vi "IPX_HTTP_Read_DI.vi"(8 "Error In":errorcluster, 9 "Voie":u16(ring) items=["1", "2", "3", "4", "5", "6", "7", "8"], 10 "Port (80-8000)":dbl=80.0, 11 "IP adress (XXX.XXX.XXX.XXX)":string) -> (0 "Error Out":errorcluster, 2 "Value":i16)   [LabVIEW 2014, in "IPX_HTTP.lvlib"]
uses:
  IPX_HTTP.lvlib
panel:
  # "Lecture des DI de la carte IPX via la lecture du status.xml"
  # "Digital Input"
  # "Please visit http://www.OpenG.org to learn about the\nOpen Source LabVIEW software movement.\n\nNOTICE -- YOU MUST LEAVE THIS NOTICE IN PLACE.  PER THE TERMS OF THE LICENSE BELOW, YOU MAY SUBLICENSE THIS SOFTWARE\nIN ANY WAY THAT DOES NOT CONFLICT WITH THIS LICENSE.\n\n### BSD License (http://www.opensource.org/licenses/bsd-license.php) Begin ###\n\nCopyright (c) 2014, Emmanuel Landrivon <emmanuel.landrivon@ircelyon.univ-lyon1.fr>\nFlorian Chapon <florian.chapon@ircelyon.univ-lyon1.fr\n\n\nAll rights reserved.\n\nRedistribution and use in source and binary forms, with or without modification, are permitted provided that the following conditions are met:\n\n    * Redistributions of source code must retain the above copyright notice, this list of conditions and the following disclaimer.\n    * Redistributions in binary form must reproduce the above copyright notice, this list of conditions and the following disclaimer in the\n       documentation and/or other materials provided with the distribution.\n  \nTHIS SOFTWARE IS PROVIDED BY THE COPYRIGHT HOLDERS AND CONTRIBUTORS \"AS IS\" AND ANY EXPRESS OR IMPLIED WARRANTIES,\nINCLUDING, BUT NOT LIMITED TO, THE IMPLIED WARRANTIES OF MERCHANTABILITY AND FITNESS FOR A PARTICULAR PURPOSE ARE\nDISCLAIMED. IN NO EVENT SHALL THE COPYRIGHT OWNER OR CONTRIBUTORS BE LIABLE FOR ANY DIRECT, INDIRECT, INCIDENTAL,\nSPECIAL, EXEMPLARY, OR CONSEQUENTIAL DAMAGES (INCLUDING, BUT NOT LIMITED TO, PROCUREMENT OF SUBSTITUTE GOODS OR\nSERVICES; LOSS OF USE, DATA, OR PROFITS; OR BUSINESS INTERRUPTION) HOWEVER CAUSED AND ON ANY THEORY OF LIABILITY,\nWHETHER IN CONTRACT, STRICT LIABILITY, OR TORT (INCLUDING NEGLIGENCE OR OTHERWISE) ARISING IN ANY WAY OUT OF THE USE\nOF THIS SOFTWARE, EVEN IF ADVISED OF THE POSSIBILITY OF SUCH DAMAGE.\n\n### BSD License End ###"
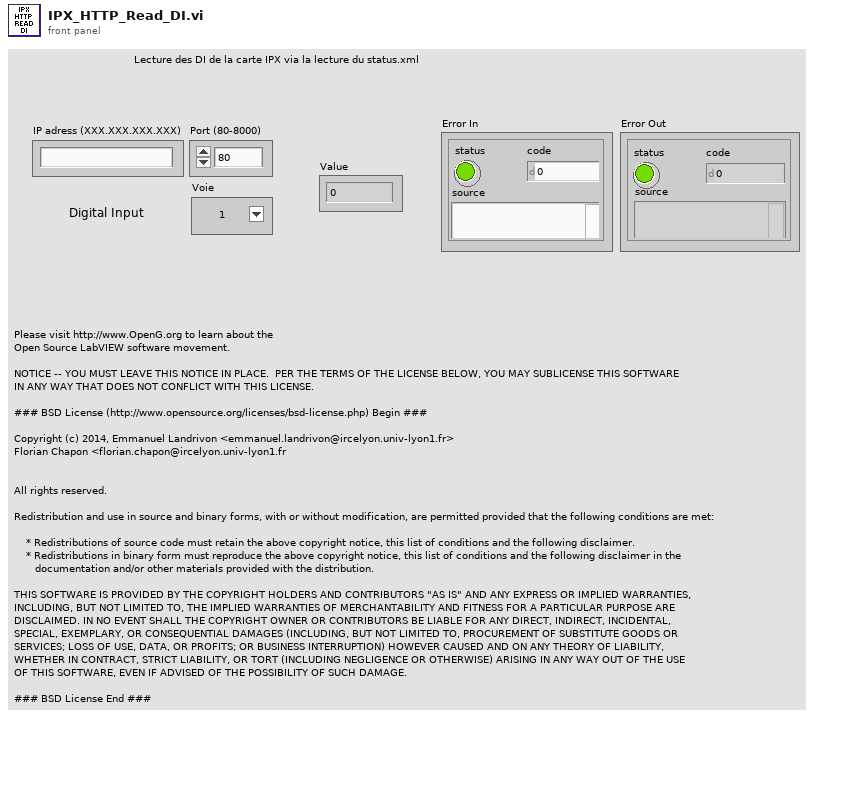
[diagram p1: front panel]
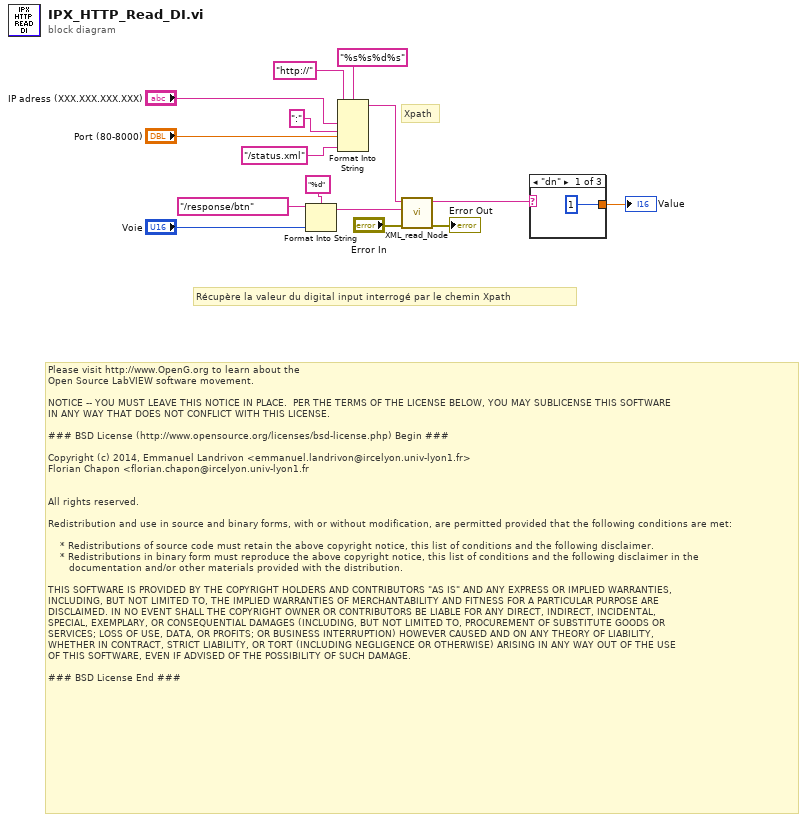
[diagram p0: block diagram]
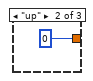
[diagram p2: hidden frame]
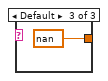
[diagram p3: hidden frame]
diagram:
  # "Please visit http://www.OpenG.org to learn about the\nOpen Source LabVIEW software movement.\n\nNOTICE -- YOU MUST LEAVE THIS NOTICE IN PLACE.  PER THE TERMS OF THE LICENSE BELOW, YOU MAY SUBLICENSE THIS SOFTWARE\nIN ANY WAY THAT DOES NOT CONFLICT WITH THIS LICENSE.\n\n### BSD License (http://www.opensource.org/licenses/bsd-license.php) Begin ###\n\nCopyright (c) 2014, Emmanuel Landrivon <emmanuel.landrivon@ircelyon.univ-lyon1.fr>\nFlorian Chapon <florian.chapon@ircelyon.univ-lyon1.fr\n\n\nAll rights reserved.\n\nRedistribution and use in source and binary forms, with or without modification, are permitted provided that the following conditions are met:\n\n    * Redistributions of source code must retain the above copyright notice, this list of conditions and the following disclaimer.\n    * Redistributions in binary form must reproduce the above copyright notice, this list of conditions and the following disclaimer in the\n       documentation and/or other materials provided with the distribution.\n  \nTHIS SOFTWARE IS PROVIDED BY THE COPYRIGHT HOLDERS AND CONTRIBUTORS \"AS IS\" AND ANY EXPRESS OR IMPLIED WARRANTIES,\nINCLUDING, BUT NOT LIMITED TO, THE IMPLIED WARRANTIES OF MERCHANTABILITY AND FITNESS FOR A PARTICULAR PURPOSE ARE\nDISCLAIMED. IN NO EVENT SHALL THE COPYRIGHT OWNER OR CONTRIBUTORS BE LIABLE FOR ANY DIRECT, INDIRECT, INCIDENTAL,\nSPECIAL, EXEMPLARY, OR CONSEQUENTIAL DAMAGES (INCLUDING, BUT NOT LIMITED TO, PROCUREMENT OF SUBSTITUTE GOODS OR\nSERVICES; LOSS OF USE, DATA, OR PROFITS; OR BUSINESS INTERRUPTION) HOWEVER CAUSED AND ON ANY THEORY OF LIABILITY,\nWHETHER IN CONTRACT, STRICT LIABILITY, OR TORT (INCLUDING NEGLIGENCE OR OTHERWISE) ARISING IN ANY WAY OUT OF THE USE\nOF THIS SOFTWARE, EVEN IF ADVISED OF THE POSSIBILITY OF SUCH DAMAGE.\n\n### BSD License End ###"
  # "Xpath"
  # "Récupère la valeur du digital input interrogé par le chemin Xpath"
  n1 = Format Into String(format string="%d", initial string="/response/btn" ("string"), "Voie") -> (resulting string=w7:string)  [unwired: 1 in, 1 out]
  n2 = Format Into String(format string="%s%s%d%s", initial string="http://", "IP adress (XXX.XXX.XXX.XXX)", ":" ("string"), "Port (80-8000)", "/status.xml" ("string")) -> (resulting string=w8:string)  [unwired: 1 in, 1 out]
  n3 = call "XML_read_Node.vi"("error in (no error)"="Error In", "Xpath adress"=w7, "Xml adress"=w8) -> ("error out"=→"Error Out":errorcluster, "Result"=w6:string)  [unwired: 7 in]
  n4 = case shown="\"dn\"" w6 {
    tunnel: [1 0 nan] -> w15
    frame "dn" {
    }
    frame "up" {
    }
    frame Default {
    }
  }
  "Value" <- w15
